vi "Bind Null.vi"(8 "error in (no error)":errorcluster, 11 "SQL Statement in":refnum<class "SQL Statement.lvclass">) -> (0 "error out":errorcluster, 2 "Unused":bool, 3 "SQL Statement out":refnum<class "SQL Statement.lvclass">)   [LabVIEW 2013, in "SQLiteSupport.lvlib" / "SQL Statement.lvclass"]
doc: "Binds a parameter as NULL. \n\nNo input value is required; the output is just to maintain compatability as a property node."
uses:
  SQL Statement.lvclass
  SQL Statement.lvclass/SQL Statement.ctl
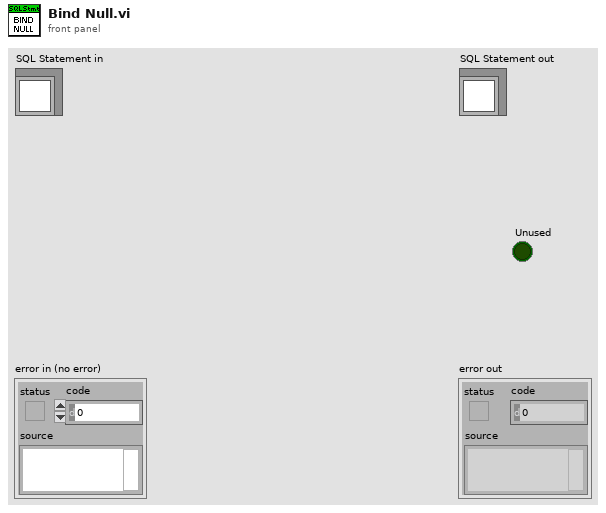
[diagram p1: front panel]
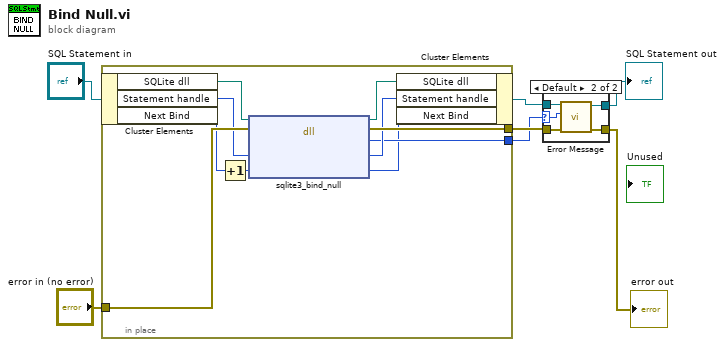
[diagram p0: block diagram]
diagram:
  n1 = in-place {
    in-place-border: "error in (no error)" -> [w17]
    in-place-border: [w16] -> w6
    in-place-border: [w9] -> w2
    n2 = in-place-cluster #1("SQL Statement in") -> ("SQLite dll"=w15:path, "Statement handle"=w12:u64, "Next Bind"=w11:i32)
    n3 = Increment(x=w11) -> (x+1=w10:i32)
    n4 = dll-call lib="C:/LabVIEW_JDP/Support/SQLite/sqlite3.dll" fn="sqlite3_bind_null"(path in=w15, error in=w17, "Statement"=w12, "Parameter"=w10) -> (path out=w14:path, error out=w16:errorcluster, "Result Code"=w9:i32, "Statement"=w13:u64, "Parameter"=w8:i32)  [unwired: 1 in]
    n5 = in-place-cluster #1("SQLite dll"=w14, "Statement handle"=w13, "Next Bind"=w8) -> (w1:refnum<class "SQL Statement.lvclass">)
  }
  n6 = case shown="Default" w2 {
    selector: w2 -> [_ w21]
    tunnel: [w18 w24] -> w5
    tunnel: w6 -> [w19 w23]
    tunnel: [w19 w22] -> w4
    tunnel: w1 -> [w18 w20]
    frame 0 {
      # "No Error"
    }
    frame Default {
      n7 = call "Error Message.vi"("error in (no error)"=w23, "error code"=w21, "SQL Statement In"=w20) -> ("error out"=w22:errorcluster, "SQL Statement Out"=w24:refnum<class "SQL Statement.lvclass">)  [unwired: 7 in]
    }
  }
  "error out" <- w4
  "SQL Statement out" <- w5
